vi "S2DS_ConfigRead sweep info (SubVI).vi"(8 "error in (no error)":errorcluster, 10 "Scan parameters in":T1 {"Y data taking" items=["in both direction", "in up direction only", "in down direction only"]; "X data taking" items=["in both direction", "in up direction only", "in down direction only"]}, 11 "Refnum in":T2) -> (0 "error out":errorcluster, 2 "Scan information (out)":T1 {"Y data taking" items=["in both direction", "in up direction only", "in down direction only"]; "X data taking" items=["in both direction", "in up direction only", "in down direction only"]}, 3 "Refnum out":T2)   [LabVIEW 2025]
uses:
  TYPE DEFS/S2DS_Sweep Info.ctl
  <vilib>/Utility/config.llb/Config Data RefNum.ctl
  <vilib>/Utility/config.llb/Read Key (U32).vi
  <vilib>/Utility/config.llb/Read Key (I32).vi
  <vilib>/Utility/config.llb/Read Key (Double).vi
  <vilib>/Utility/config.llb/Read Key (Boolean).vi
  <vilib>/Utility/config.llb/Read Key (String).vi
  <vilib>/Utility/config.llb/NI_LVConfig.lvlib
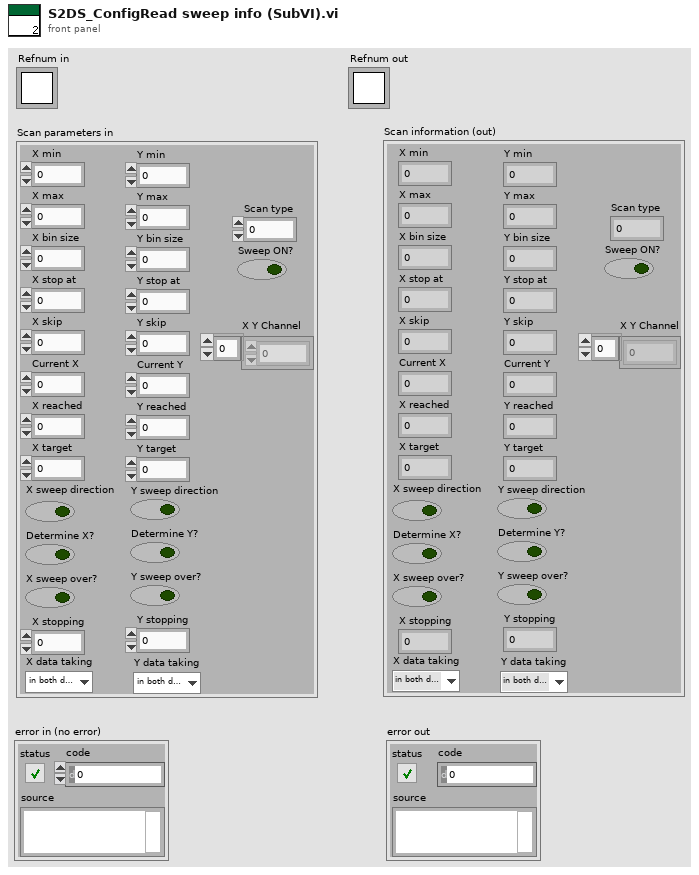
[diagram p1: front panel]
types:
  T1 = typedef "S2DS_Sweep Info.ctl" = cluster{"X min":ext, "X max":dbl, "Y min":dbl, "Y max":dbl, "X bin size":dbl, "Y bin size":dbl, "X stop at":dbl, "Y stop at":dbl, "X skip":u64, "Y skip":u64, "Current X":dbl, "Current Y":dbl, "X reached":i32, "Y reached":i32, "X target":dbl, "Y target":dbl, "Sweep ON?":bool, "X sweep direction":bool, "Y sweep direction":bool, "Determine X?":bool, "Determine Y?":bool, "X sweep over?":bool, "Y sweep over?":bool, "Scan type":i32, "X stopping":i32, "Y stopping":i32, "X Y Channel":u16[], "X data taking":u16, "Y data taking":u16}
  T2 = typedef "NI_LVConfig.lvlib/Config Data RefNum.ctl" = refnum<k1>
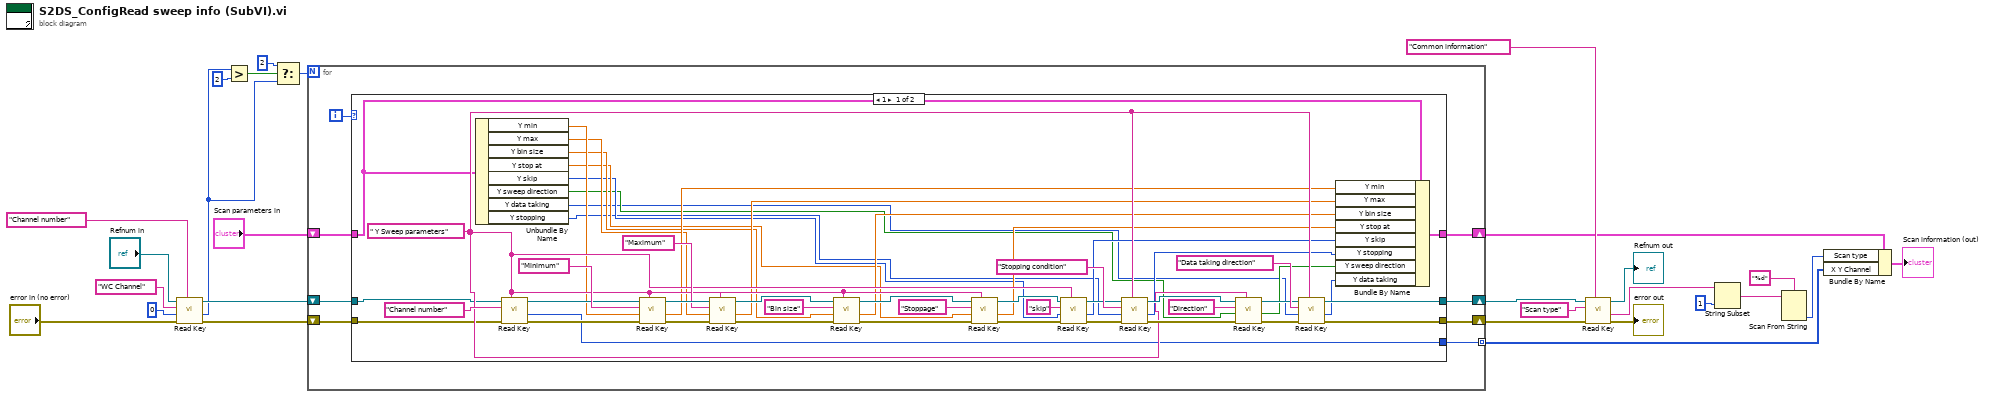
[diagram p0: block diagram]
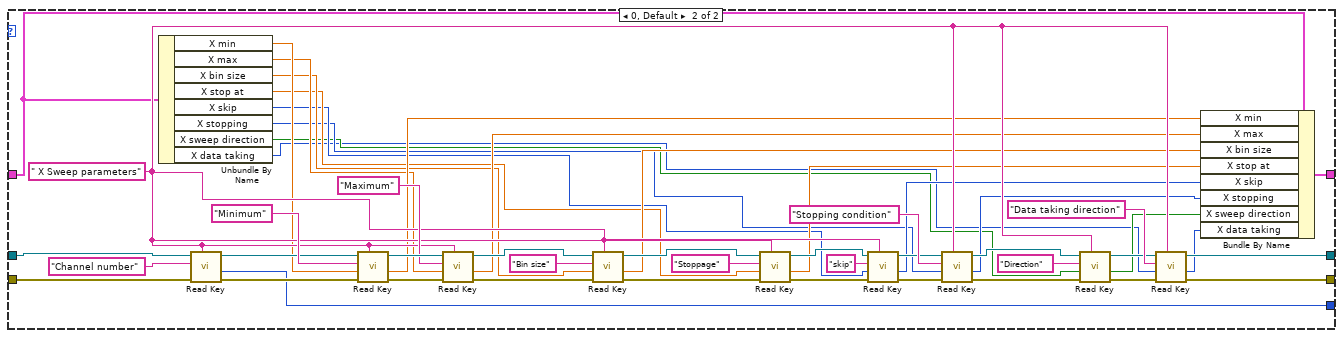
[diagram p2: hidden frame]
diagram:
  n1 = call-poly <vilib>:"Read Key.vi"("section"="Channel number", "error in (no error)"="error in (no error)", "default value"=u32 0, "key"="WC Channel", "refnum"="Refnum in") -> ("error out"=w15:errorcluster, "value"=w4:u32, "refnum out"=w14:T2)  [unwired: 4 out]
  n2 = Greater?(x=w4, y=u32 2) -> (0:w5:bool)
  n3 = Select(t=u32 2, s=w5, f=w4) -> (s? t:f=w2:u32)
  n4 = for {
    N: w2 -> [_]
    shift-right: [w32] -> w23
    shift-left: w14 -> [w33]
    shift-right: [w31] -> w25
    shift-left: w15 -> [w34]
    tunnel: [w29] -> w7 mode=indexing
    shift-right: [w28] -> w1
    shift-left: "Scan parameters in" -> [w35]
    i -> [w30]
    n5 = case shown="1" w30 {
      tunnel: w35 -> [w44 w93]
      tunnel: [w61 w110] -> w32
      tunnel: [w62 w111] -> w31
      tunnel: w33 -> [w58 w107]
      tunnel: w34 -> [w56 w105]
      tunnel: [w54 w103] -> w29
      tunnel: [w45 w94] -> w28
      frame 1 {
        w59 = " Y Sweep parameters"
        n6 = Unbundle By Name(w44) -> ("Y min"=w43:dbl, "Y max"=w42:dbl, "Y bin size"=w41:dbl, "Y stop at"=w40:dbl, "Y skip"=w39:u64, "Y sweep direction"=w38:bool, "Y data taking"=w37:u16, "Y stopping"=w36:i32)
        n7 = call-poly <vilib>:"Read Key.vi"("section"=w59, "error in (no error)"=w56, "key"="Channel number", "refnum"=w58) -> ("error out"=w55:errorcluster, "value"=w54:i32, "refnum out"=w57:T2)  [unwired: 4 in, 1 out]
        n8 = call-poly <vilib>:"Read Key.vi"("section"=w59, "error in (no error)"=w55, "default value"=w43, "key"="Minimum", "refnum"=w57) -> ("error out"=w83:errorcluster, "value"=w53:dbl, "refnum out"=w81:T2)  [unwired: 3 in, 1 out]
        n9 = call-poly <vilib>:"Read Key.vi"("section"=w59, "error in (no error)"=w83, "default value"=w42, "key"="Maximum", "refnum"=w81) -> ("error out"=w84:errorcluster, "value"=w52:dbl, "refnum out"=w82:T2)  [unwired: 3 in, 1 out]
        n10 = call-poly <vilib>:"Read Key.vi"("section"=w59, "error in (no error)"=w84, "default value"=w41, "key"="Bin size", "refnum"=w82) -> ("error out"=w66:errorcluster, "value"=w51:dbl, "refnum out"=w67:T2)  [unwired: 3 in, 1 out]
        n11 = call-poly <vilib>:"Read Key.vi"("section"=w59, "error in (no error)"=w66, "default value"=w40, "key"="Stoppage", "refnum"=w67) -> ("error out"=w70:errorcluster, "value"=w50:dbl, "refnum out"=w73:T2)  [unwired: 3 in, 1 out]
        n12 = call-poly <vilib>:"Read Key.vi"("section"=w59, "error in (no error)"=w70, "default value"=w39, "key"="skip", "refnum"=w73) -> ("error out"=w69:errorcluster, "value"=w49:i32, "refnum out"=w72:T2)  [unwired: 3 in, 1 out]
        n13 = call-poly <vilib>:"Read Key.vi"("section"=w59, "error in (no error)"=w69, "default value"=w36, "key"="Stopping condition", "refnum"=w72) -> ("error out"=w68:errorcluster, "value"=w48:i32, "refnum out"=w71:T2)  [unwired: 3 in, 1 out]
        n14 = call-poly <vilib>:"Read Key.vi"("section"=w59, "error in (no error)"=w68, "default value"=w38, "key"="Direction", "refnum"=w71) -> ("error out"=w63:errorcluster, "value"=w47:bool, "refnum out"=w64:T2)  [unwired: 3 in, 1 out]
        n15 = call-poly <vilib>:"Read Key.vi"("section"=w59, "error in (no error)"=w63, "default value"=w37, "key"="Data taking direction", "refnum"=w64) -> ("error out"=w62:errorcluster, "value"=w46:i32, "refnum out"=w61:T2)  [unwired: 3 in, 1 out]
        n16 = Bundle By Name(cluster=w44, "Y min"=w53, "Y max"=w52, "Y bin size"=w51, "Y stop at"=w50, "Y skip"=w49, "Y stopping"=w48, "Y sweep direction"=w47, "Y data taking"=w46) -> (w45:T1)
      }
      frame 0, Default {
        w108 = " X Sweep parameters"
        n17 = Unbundle By Name(w93) -> ("X min"=w92:ext, "X max"=w91:dbl, "X bin size"=w90:dbl, "X stop at"=w89:dbl, "X skip"=w88:u64, "X stopping"=w87:i32, "X sweep direction"=w86:bool, "X data taking"=w85:u16)
        n18 = call-poly <vilib>:"Read Key.vi"("section"=w108, "error in (no error)"=w105, "key"="Channel number", "refnum"=w107) -> ("error out"=w104:errorcluster, "value"=w103:i32, "refnum out"=w106:T2)  [unwired: 4 in, 1 out]
        n19 = call-poly <vilib>:"Read Key.vi"("section"=w108, "error in (no error)"=w104, "default value"=w92, "key"="Minimum", "refnum"=w106) -> ("error out"=w132:errorcluster, "value"=w102:dbl, "refnum out"=w130:T2)  [unwired: 3 in, 1 out]
        n20 = call-poly <vilib>:"Read Key.vi"("section"=w108, "error in (no error)"=w132, "default value"=w91, "key"="Maximum", "refnum"=w130) -> ("error out"=w133:errorcluster, "value"=w101:dbl, "refnum out"=w131:T2)  [unwired: 3 in, 1 out]
        n21 = call-poly <vilib>:"Read Key.vi"("section"=w108, "error in (no error)"=w133, "default value"=w90, "key"="Bin size", "refnum"=w131) -> ("error out"=w115:errorcluster, "value"=w100:dbl, "refnum out"=w116:T2)  [unwired: 3 in, 1 out]
        n22 = call-poly <vilib>:"Read Key.vi"("section"=w108, "error in (no error)"=w115, "default value"=w89, "key"="Stoppage", "refnum"=w116) -> ("error out"=w119:errorcluster, "value"=w99:dbl, "refnum out"=w122:T2)  [unwired: 3 in, 1 out]
        n23 = call-poly <vilib>:"Read Key.vi"("section"=w108, "error in (no error)"=w119, "default value"=w88, "key"="skip", "refnum"=w122) -> ("error out"=w118:errorcluster, "value"=w98:i32, "refnum out"=w121:T2)  [unwired: 3 in, 1 out]
        n24 = call-poly <vilib>:"Read Key.vi"("section"=w108, "error in (no error)"=w118, "default value"=w87, "key"="Stopping condition", "refnum"=w121) -> ("error out"=w117:errorcluster, "value"=w97:i32, "refnum out"=w120:T2)  [unwired: 3 in, 1 out]
        n25 = call-poly <vilib>:"Read Key.vi"("section"=w108, "error in (no error)"=w117, "default value"=w86, "key"="Direction", "refnum"=w120) -> ("error out"=w112:errorcluster, "value"=w96:bool, "refnum out"=w113:T2)  [unwired: 3 in, 1 out]
        n26 = call-poly <vilib>:"Read Key.vi"("section"=w108, "error in (no error)"=w112, "default value"=w85, "key"="Data taking direction", "refnum"=w113) -> ("error out"=w111:errorcluster, "value"=w95:i32, "refnum out"=w110:T2)  [unwired: 3 in, 1 out]
        n27 = Bundle By Name(cluster=w93, "X min"=w102, "X max"=w101, "X bin size"=w100, "X stop at"=w99, "X skip"=w98, "X stopping"=w97, "X sweep direction"=w96, "X data taking"=w95) -> (w94:T1)
      }
    }
  }
  n28 = call-poly <vilib>:"Read Key.vi"("section"="Common information", "error in (no error)"=w25, "key"="Scan type", "refnum"=w23) -> ("error out"=→"error out":errorcluster, "value"=w12:string, "refnum out"=→"Refnum out":T2)  [unwired: 4 in, 1 out]
  n29 = String Subset(string=w12, length (rest)=1 ("length (rest)")) -> (substring=w10:string)  [unwired: 1 in]
  n30 = Scan From String(format string="%d", input string=w10) -> (output 1=w8:i32)  [unwired: 3 in, 3 out]
  n31 = Bundle By Name(cluster=w1, "Scan type"=w8, "X Y Channel"=w7) -> (→"Scan information (out)":T1)
